vi "discover channels.vi"(8 "error in":errorcluster, 10 "module configuration":refnum<class "TBM module configuration.lvclass">, 11 "module in":refnum<class "Scan Engine runtime.lvclass">) -> (0 "error out":errorcluster, 2 "updated configuration":refnum<class "TBM module configuration.lvclass">, 3 "module out":refnum<class "Scan Engine runtime.lvclass">)   [LabVIEW 2013, in "Scan Engine runtime.lvclass"]
doc: "Provides an interface for discovering channels at runtime. While this interface performs no operations, a child should provide an override which performs discovery of any channel information that may be available at run time and not at configure time."
uses:
  Scan Engine runtime.lvclass
  <vilib>/NI/Tag Bus Module Framework/module configuration/TBM module configuration.lvclass
  configuration/Scan Engine configuration.lvclass
  configuration/Scan Engine configuration.lvclass/Scan Engine configuration.ctl
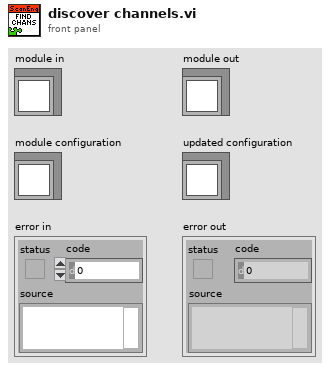
[diagram p1: front panel]
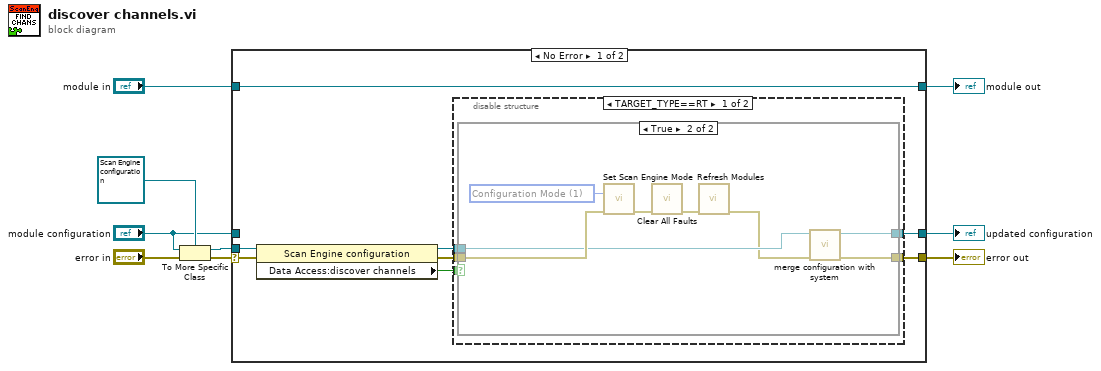
[diagram p0: block diagram]
diagram:
  n1 = To More Specific Class(target class=refnum<class "Scan Engine configuration.lvclass"> refnum ("Scan Engine configuration"), reference="module configuration", error in="error in") -> (specific class reference=w1:refnum<class "Scan Engine configuration.lvclass">, error out=w7:errorcluster)
  n2 = case shown="No Error" w7 {
    selector: w7 -> [w17 w36]
    tunnel: "module in" -> [w15 w37]
    tunnel: [w15 w37] -> w5
    tunnel: [w10 w36] -> w4
    tunnel: "module configuration" -> [_ w35]
    tunnel: [w13 w35] -> w2
    tunnel: w1 -> [w16 _]
    frame No Error {
      n3 = property class="Scan Engine configuration"(reference=w16, error in=w17) -> (reference out=w12:refnum<class "Scan Engine configuration.lvclass">, error out=w11:errorcluster, "Data Access:discover channels"=w14:bool)
      n4 = disable-structure shown="TARGET_TYPE==RT" {
        disable-tunnel: w14 -> [w22 _]
        disable-tunnel: [w21 w34] -> w13
        disable-tunnel: w12 -> [w20 w34]
        disable-tunnel: w11 -> [w19 w33]
        disable-tunnel: [w18 w33] -> w10
        frame condition #0 {
          n5 = case shown="True" w22 {
            tunnel: [w24 w30] -> w21
            tunnel: w20 -> [w24 w31]
            tunnel: w19 -> [w23 w32]
            tunnel: [w23 w29] -> w18
            frame False {
            }
            frame True {
              w28 = 1 items=["Configuration Mode"=1, "Active Mode"=2] ("mode (Active Mode)")
              n6 = call <vilib>:"Set Scan Engine Mode.vi"("mode (Active Mode)"=w28, "error in (no error)"=w32) -> ("error out"=w26:errorcluster)  [unwired: 13 in]
              n7 = call <vilib>:"Clear All Faults.vi"("error in (no error)"=w26) -> ("error out"=w25:errorcluster)  [unwired: 10 in]
              n8 = call <vilib>:"Refresh Modules.vi"("error in (no error)"=w25) -> ("error out"=w27:errorcluster)  [unwired: 10 in]
              n9 = call "merge configuration with system.vi"("error in"=w27, "Scan Engine configuration in"=w31) -> ("error out"=w29:errorcluster, "Scan Engine configuration out"=w30:refnum<class "Scan Engine configuration.lvclass">)  [unwired: 8 in]
            }
          }
        }
        frame condition #1 (active) {
        }
      }
    }
    frame Error {
    }
  }
  "error out" <- w4
  "module out" <- w5
  "updated configuration" <- w2
